vi "Set Binding.vi"(11 "Recipes.Binding":T1) -> (3 "concatenated string":string)   [LabVIEW 2014, in "Programing Logic.lvclass"]
uses:
  Programming Logic/Programing Logic.lvclass
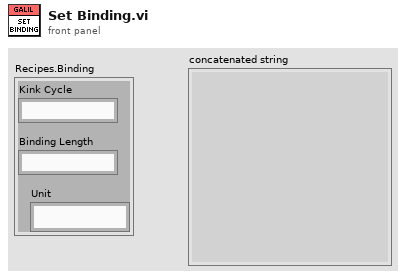
[diagram p1: front panel]
types:
  T1 = cluster{"Kink Cycle":string, "Binding Length":string, "Unit":string}
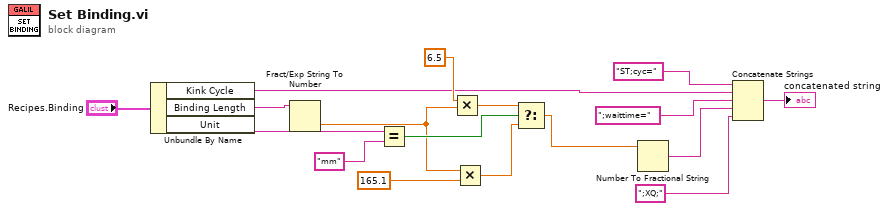
[diagram p0: block diagram]
diagram:
  n1 = Unbundle By Name("Recipes.Binding") -> ("Kink Cycle"=w3:string, "Binding Length"=w2:string, "Unit"=w15:string)
  n2 = Fract/Exp String To Number(string=w2) -> (number=w1:dbl)  [unwired: 3 in, 1 out]
  n3 = Equal?(x=w15, y="mm") -> (x = y?=w6:bool)
  n4 = Multiply(x=6.5, y=w1) -> (x*y=w9:dbl)
  n5 = Multiply(x=w1, y=165.1) -> (x*y=w4:dbl)
  n6 = Select(t=w9, s=w6, f=w4) -> (s? t:f=w7:dbl)
  n7 = Number To Fractional String(number=w7) -> (F-format string=w8:string)  [unwired: 3 in]
  n8 = Concatenate Strings("ST;cyc=" ("string"), w3, ";waittime=" ("string"), w8, ";XQ;" ("string")) -> (→"concatenated string":string)
